vi "slow_control_2_01.vi"() -> ()   [LabVIEW 2018]
uses:
  <vilib>/DAQmx/read.llb/DAQmx Read (Analog 1D DBL NChan 1Samp).vi
  <vilib>/DAQmx/create/channels.llb/DAQmx Create Channel (AI-Voltage-Basic).vi
  <vilib>/DAQmx/miscellaneous.llb/DAQmx Fill In Error Info.vi
  <instrlib>/Lake Shore 335/Lake Shore 335.lvlib
  <instrlib>/CAEN PSM/CAEN PSM.lvlib
panel:
  out "Coldhead":dbl
  out "Heater":dbl
  out "Cycle number":i32
  out "TOBA tester":dbl[][](array[numeric])
  in  "Cycles to execute":dbl=5.0 format="%#_13g"
  out "Moving average Det. P":dbl
  in  "N samples":i32=20
  in  "Allows tabs on \nfront panel":T1(tab)
  in  "Flow meter is AI number:":enum16{"0", "1", "2", "3", "4", "5", "6", "7"}(ring)=enum."3"
  in  "Detector Pressure is AI number:":enum16{"0", "1", "2", "3", "4", "5", "6", "7"}(ring)
  in  "physical channels":tag[](array[tag])=["9207/ai0", "9207/ai1", "9207/ai2", "9207/ai3", "9207/ai4", "9207/ai5", "9207/ai6", "9207/ai7"]
  in  "input terminal configurations":i32[](array[ring]) items=["Default"=-1, "RSE"=10083, "NRSE"=10078, "Differential"=10106, "Pseudodifferential"=12529]
  in  "Heater range":u16(ring) items=["Off", "Low (On)", "Medium", "High"]
  in  "Setpoint (°C)":dbl=-100.0 format="%.1f"
  in  "PID settings":cluster{"P":dbl, "I":dbl, "D":dbl}={"P"=50.0, "I"=20.0, "D"=120.0}
  in  "COM-port LakeShore":refnum<visa-resource-name>
  in  "ID Query":bool=TRUE
  in  "COM-port CAEN 1":refnum<visa-resource-name>
  in  "COM-port CAEN 2":refnum<visa-resource-name>
  out "Heater power (%) 2":cluster{timestamp[], dbl[]}[](graph)
  out "Temp B":dbl
  out "Temp A":dbl
  out "LakeShore readings 2":dbl[](array[numeric])
  out "Raw P (Volt)":dbl[](array[numeric]) format="%0.4f"
  in  "T 20":bool
  in  "T 19":bool
  in  "T 18":bool
  in  "T 17":bool
  in  "T 16":bool
  in  "T 15":bool
  in  "Detector P":bool
  in  "Overpressure threshold":dbl
  in  "Underpressure threshold":dbl
  out "Comm. status":bool
  in  "High Temp threshold":dbl format="%#_13g"
  in  "Low Temp threshold":dbl format="%#_13g"
  in  "Ignore Initialization Errors":bool caption="Ignore init. errors?"
  out "LakeShore status":bool
  out "NI mod1 (P) status":bool
  out "CAEN 1 status":bool
  out "CAEN 2 status":bool
  out "Initialization status":bool
  out "Heater power (%)":cluster{timestamp[], dbl[]}[](graph)
  out "Flow (SLPM)":cluster{timestamp[], dbl[]}[](graph)
  out "Pressure":cluster{timestamp[], dbl[]}[](graph)
  out "Phase Diagram":cluster{"X":dbl, "Y":dbl}[](graph)
  in  "Temp. Channel selector":string(combo)="Average 15 to 20"
  out "Temperature":cluster{timestamp[], dbl[]}[](graph)
  in  "N samples":i32=30
  out "Average Flow (SLPM)":dbl caption="Average Flow (SLPM), of"
  in  "Pause?":bool
  out "Integrated Flow (SL)":dbl
  in  "Reset?":bool
  out "LakeShore readings":dbl[](array[numeric])
  out "Temp. 1":dbl
  out "Temp. 2":dbl
  out "Temp. 3":dbl
  out "Temp. 4":dbl
  out "Temp. 5":dbl
  out "Temp. 6":dbl
  out "Temp. 7":dbl
  out "Temp. 8":dbl
  out "Temp. 9":dbl
  out "Temp. 10":dbl
  out "Temp. 11":dbl
  out "Temp. 12":dbl
  out "Temp. 13":dbl
  out "Temp. 14":dbl
  out "Temp. 15":dbl
  out "Temp. 16":dbl
  out "Temp. 17":dbl
  out "Temp. 18":dbl
  out "Temp. 19":dbl
  out "Temp. 20":dbl
  out "1 to 4":dbl[](array[numeric])
  out "5 to 8":dbl[](array[numeric])
  out "9 to 12":dbl[](array[numeric])
  out "13 to 16":dbl[](array[numeric])
  out "17 to 20":dbl[](array[numeric])
  in  "Temperature Channel selector":string(combo)="Average 15 to 20"
  out "Historical Large Phase Diagram":cluster{dbl[], dbl[]}[](graph)
  out "Large Phase Diagram":cluster{"X":dbl, "Y":dbl}[](graph)
  in  "Temperature Channel selector":string(combo)="Average 15 to 20"
  in  "Set to zero":bool
  out "Bottom gate":dbl(knob) scale=0.0..-3000.0
  out "Top gate":dbl(knob) scale=0.0..3000.0
  in  "Apply Voltage":bool
  in  "VSet (V)":dbl[](array[numeric])
  in  "IMax (uA)":dbl[](array[numeric])
  in  "VMax (V)":dbl[](array[numeric])
  out "Cathode":dbl(knob) scale=0.0..-5000.0
  out "Anode":dbl(knob) scale=0.0..4000.0
  out "PMT 2":dbl(knob) scale=0.0..1000.0
  out "PMT 1":dbl(knob) scale=1.0..1000.0
  out "Vmon (V)":dbl[](array[numeric])
  out "IMon (uA)":dbl[](array[numeric])
  in  "Read V every N cycles":i16=120
  in  "Reset anode":bool
  in  "Kill every Y minutes":i32=10
  in  "Keep off for X seconds":i32=10
  out "?":bool
  out "Killed":bool
  out "Restarted":bool
  out "Anode times":dbl[](array[numeric]) format="%_12f"
  out "Anode times 2":timestamp[](array[timestamp])
  in  "Kill voltage":bool
  in  "stop":bool
  out "Voltages":dbl[](array[numeric])
  out "Started up?":bool
  out "TOBA appended":dbl[][](array[numeric])
  in  "Read T every N cycles":i32=2
  out "Time until next cycle":dbl format="%.3g"
  in  "Time per cycle (s)":i32=2 caption="Time Target (s)"
  # "<- Proof of concept for New/Old T + New P"
  # "PMT 1"
  # "PMT 2"
  # "Anode"
  # "Cathode"
  # "Top gate"
  # "Bottom gate"
  # "Connection settings"
  # "Lakeshore settings"
  # "NI 9207 settings"
  # "Gain (P) (XX.X)"
  # "Reset (I) (XX.X)"
  # "Rate (D) (X.X%)"
  # "Specify inputs:"
  # "Heater tests"
  # "Move to Quick Temp tab ^"
  # "Alarm indicators"
  # "Thresholds"
  # "Alarm conditions"
  # "CAEN 1"
  # "Data"
  # "PMT 1"
  # "PMT 1"
  # "PMT 2"
  # "PMT 2"
  # "Anode"
  # "Anode"
  # "Cathode"
  # "Cathode"
  # "Top gate"
  # "Top gate"
  # "Bottom gate"
  # "Bottom gate"
  # "Settings"
  # "PMT 1"
  # "PMT 1"
  # "PMT 2"
  # "PMT 2"
  # "Anode"
  # "Anode"
  # "Cathode"
  # "Cathode"
  # "Top gate"
  # "Top gate"
  # "Bottom gate"
  # "Bottom gate"
  # "CAEN 2"
  # "PMT 1"
  # "PMT 2"
  # "Anode"
  # "Cathode"
  # "Needle gauges or other displays go here"
  # "Top gate"
  # "Bottom gate"
  # "Time of last reset"
  # "Time of last reactivation"
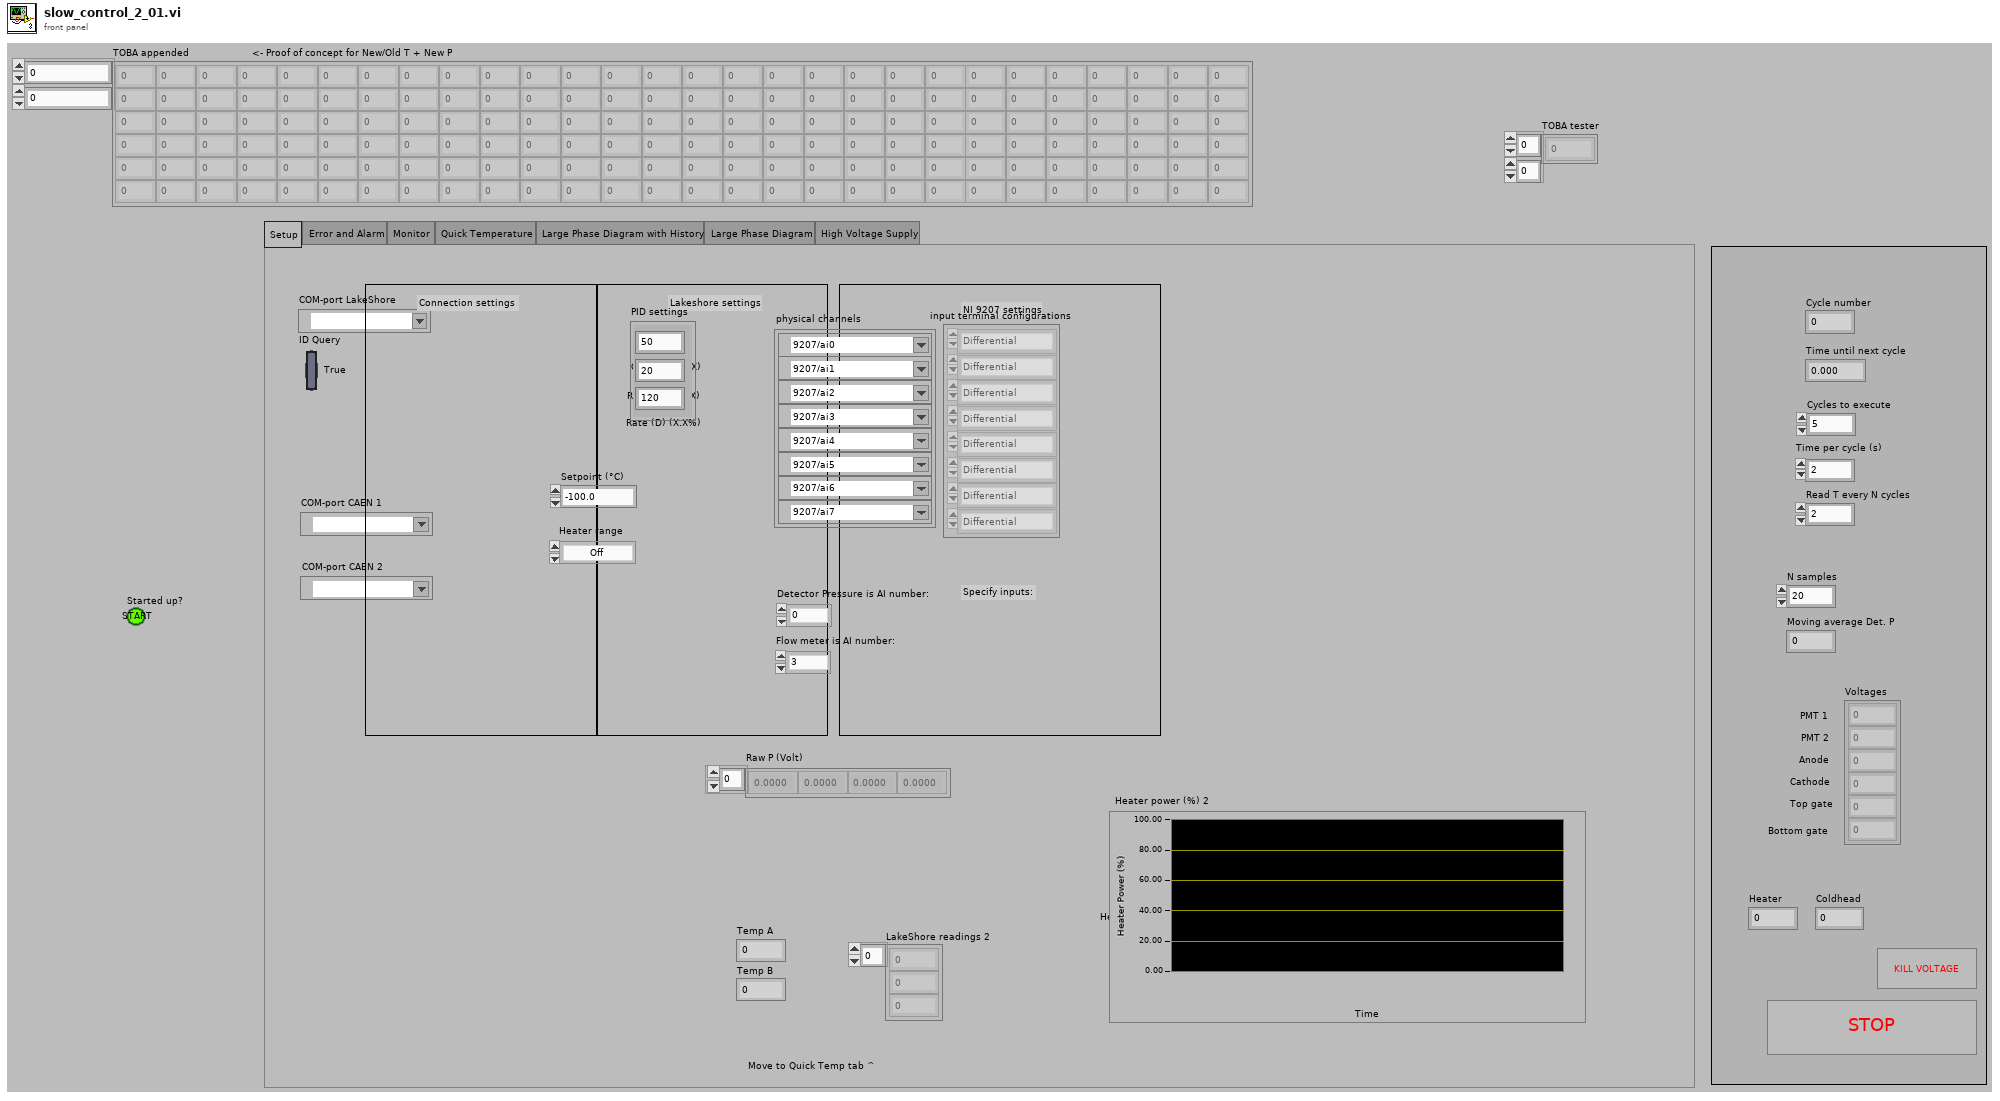
[diagram p1: front panel]
types:
  T1 = enum32{"Setup", "Error and Alarm", "Monitor", "Quick Temperature", "Large Phase Diagram with History", "Large Phase Diagram", "High Voltage Supply"}
  T2 = cluster{"Baud Rate":u32, "Parity":u16, "Data Bits":u16, "Stop Bits":u16, "Flow Control":u16}
  T3 = cluster{"VISA resource name out":refnum<visa-resource-name>, "error out":errorcluster}
  T4 = cluster{"task out":refnum<k21>, "error out":errorcluster}
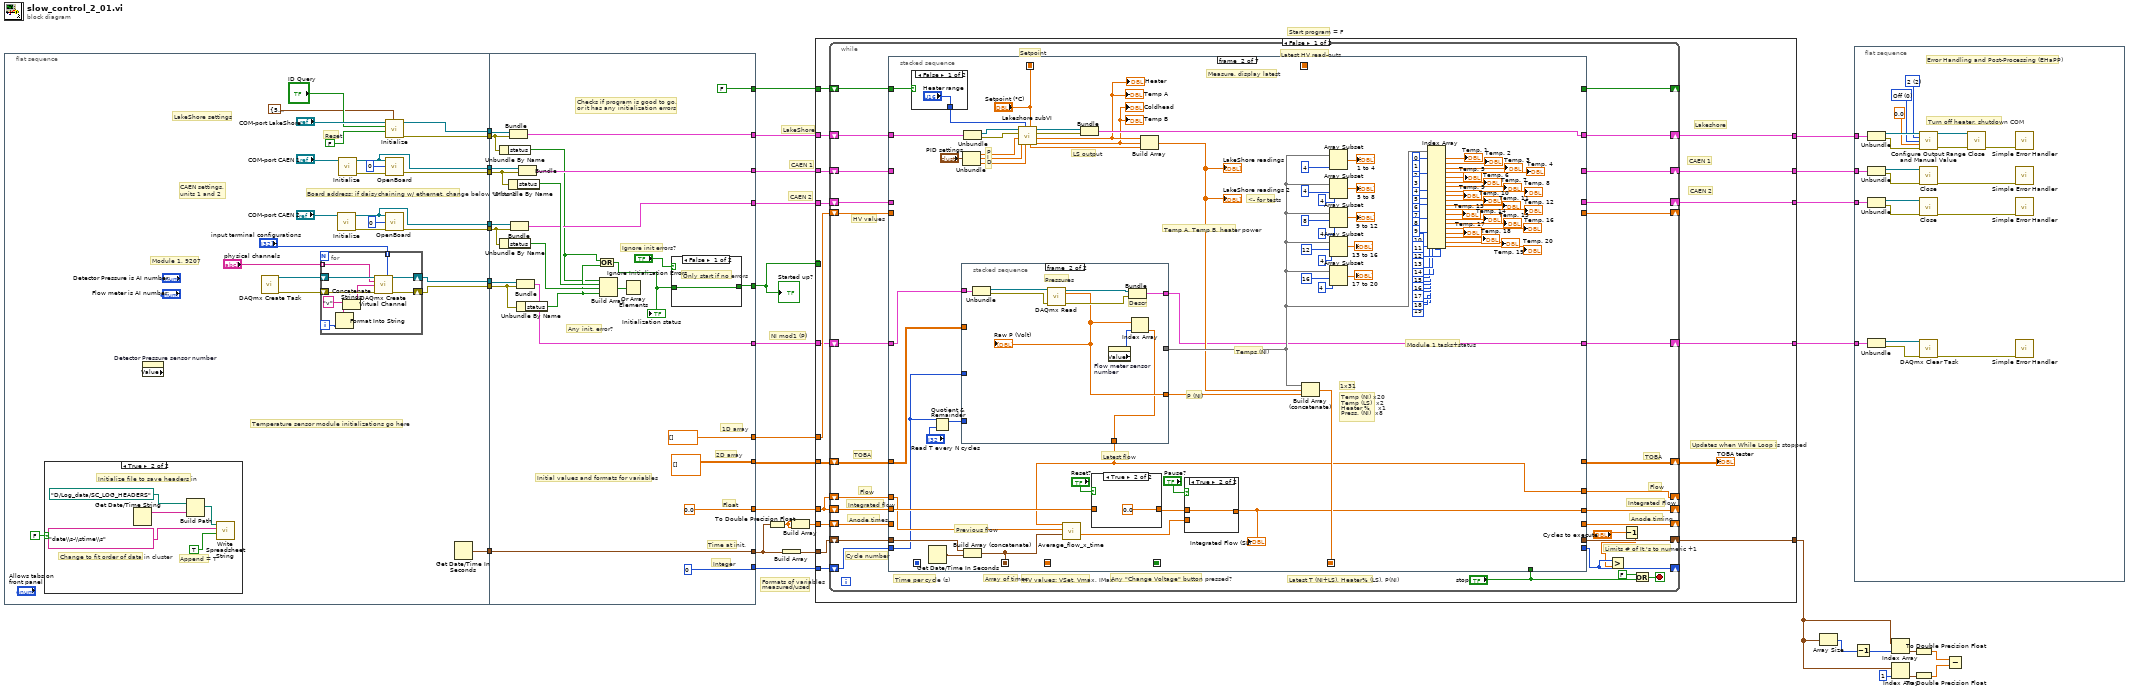
[diagram p0: block diagram]
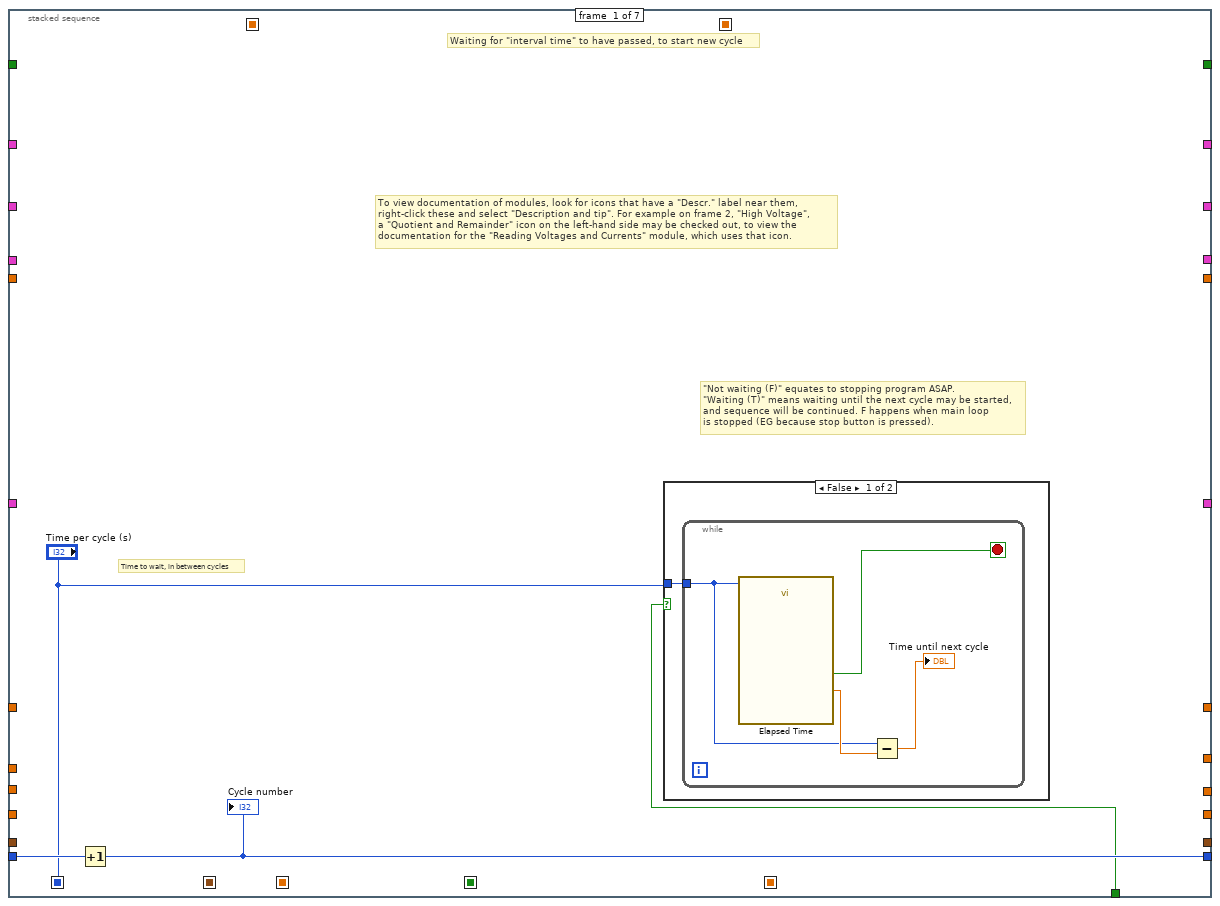
[diagram p2: hidden frame]
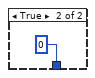
[diagram p4: hidden frame]
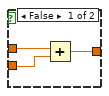
[diagram p6: hidden frame]
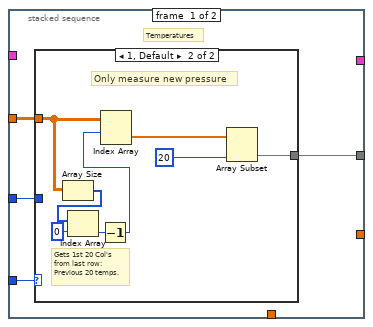
[diagram p7: hidden frame]
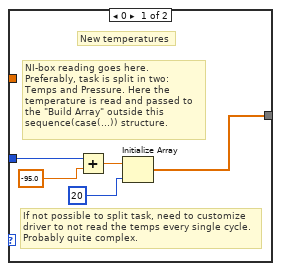
[diagram p8: hidden frame]
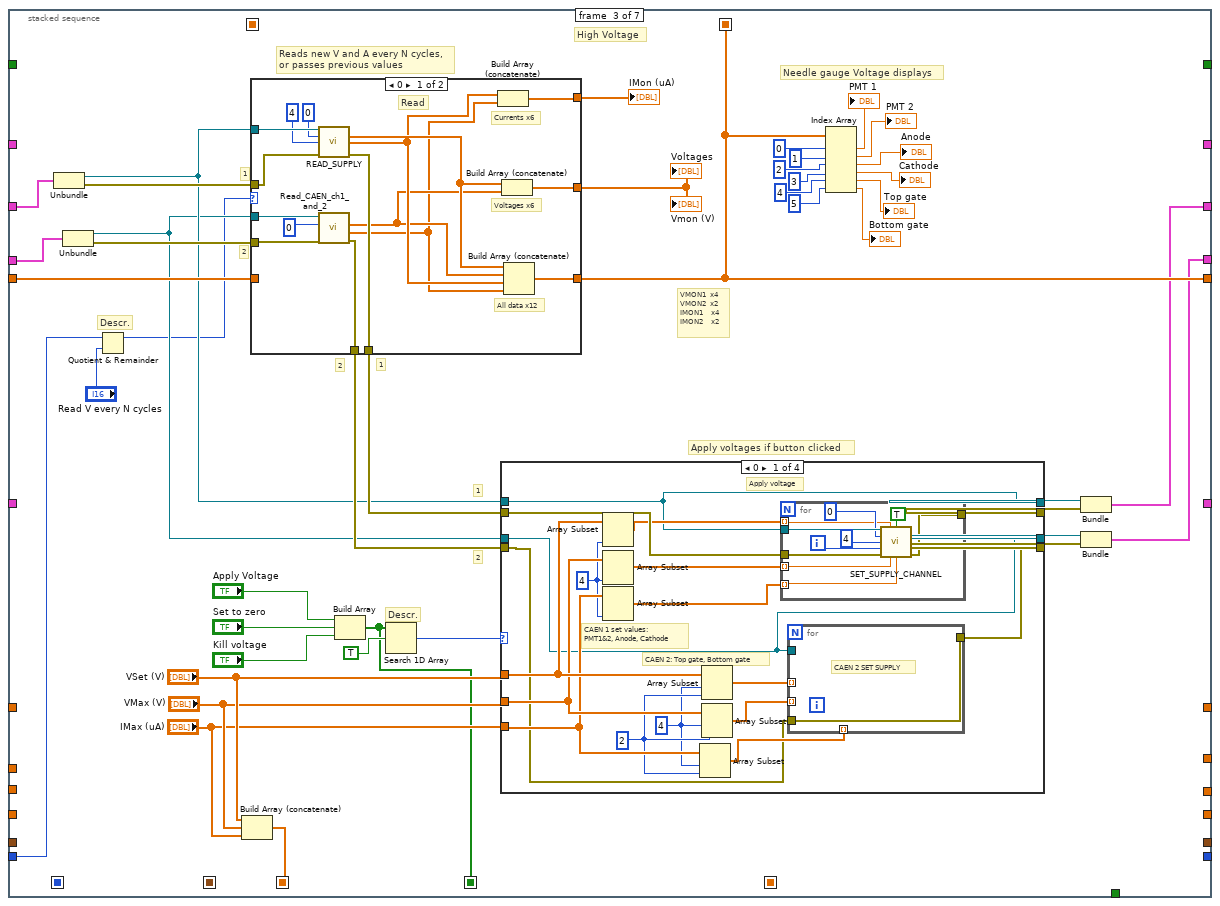
[diagram p9: hidden frame]
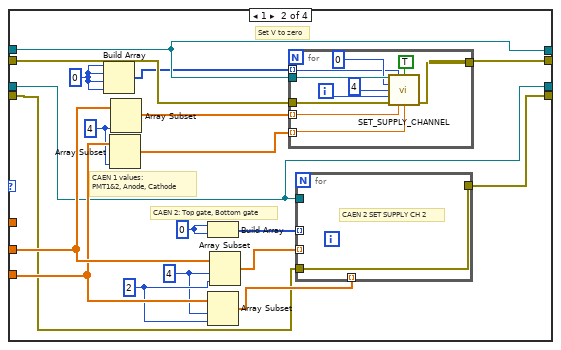
[diagram p10: hidden frame]
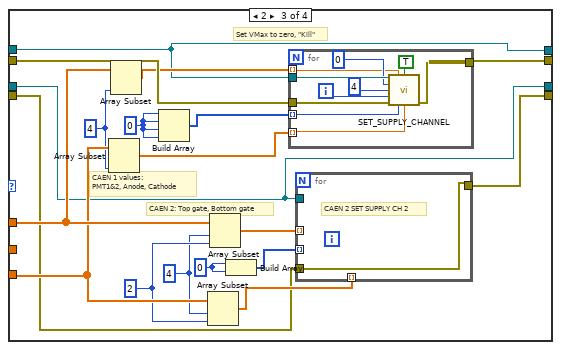
[diagram p11: hidden frame]
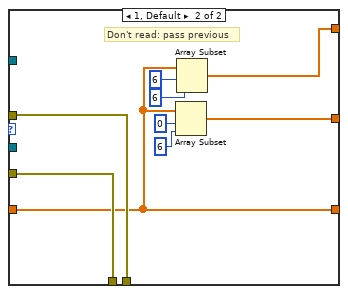
[diagram p13: hidden frame]
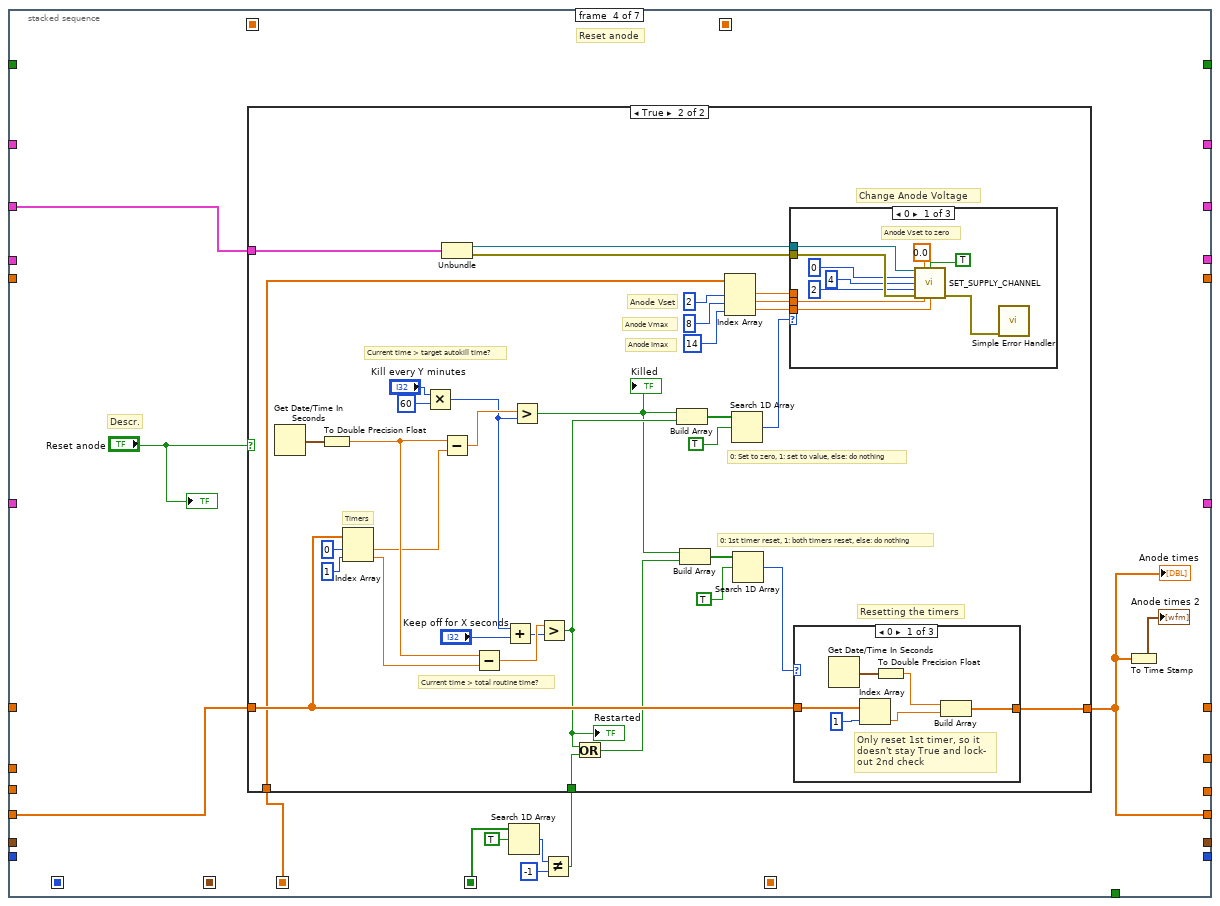
[diagram p14: hidden frame]
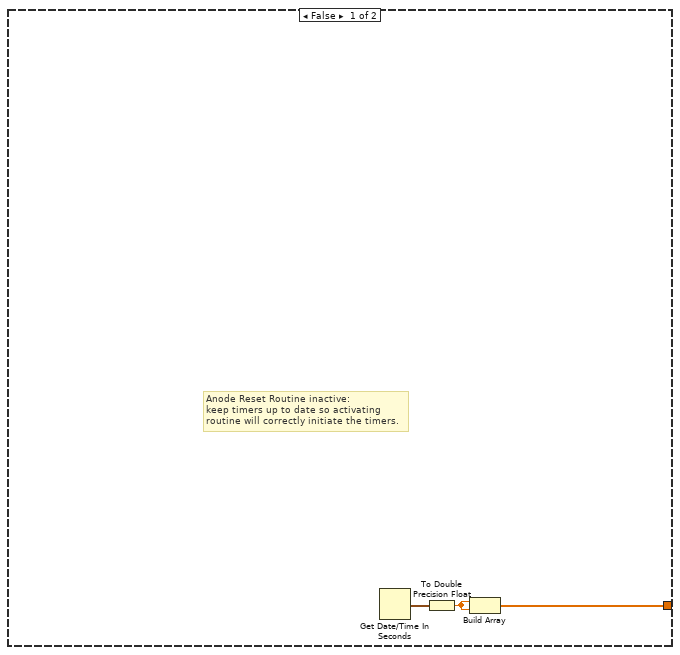
[diagram p15: hidden frame]
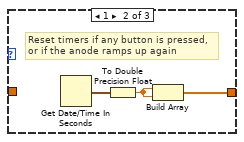
[diagram p16: hidden frame]
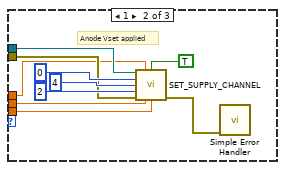
[diagram p18: hidden frame]
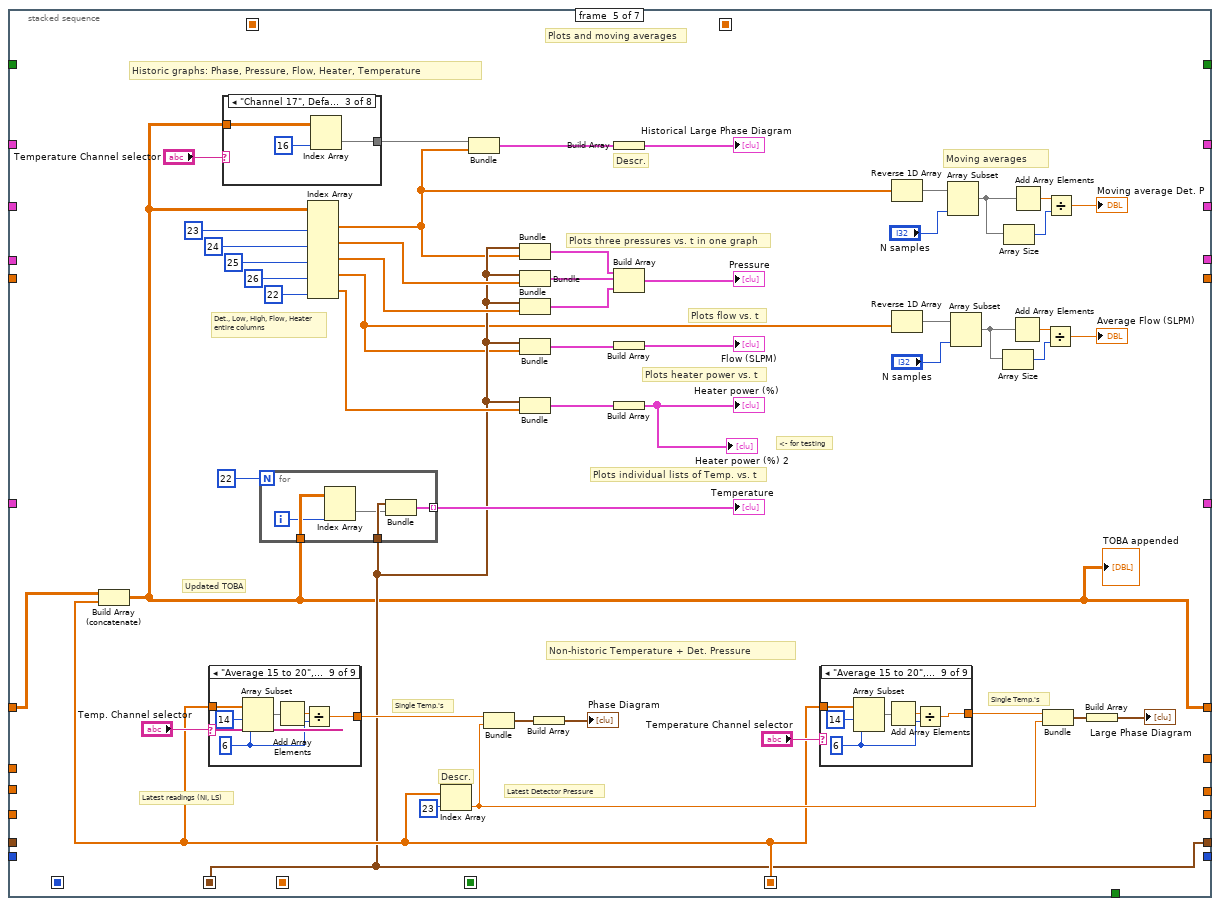
[diagram p20: hidden frame]
diagram:
  # "NI mod1 (P)"
  # "Start program = F"
  # "CAEN 2"
  # "CAEN 1"
  # "LakeShore"
  # "Formats of variables\nmeasured/used"
  n1 = flat-sequence {
    tunnel: [w56] -> w35
    tunnel: [w55] -> w34
    tunnel: [w42] -> w33
    tunnel: [w52] -> w32
    tunnel: [w39] -> w31
    tunnel: [w51] -> w25
    tunnel: [w47] -> w15
    tunnel: [w46] -> w14
    tunnel: [w40] -> w5
    tunnel: w35 -> [w97]
    tunnel: w34 -> [w96]
    tunnel: w33 -> [w94]
    tunnel: w32 -> [w93]
    tunnel: w31 -> [w83]
    tunnel: [w98] -> w12
    tunnel: [0.0] -> w11
    tunnel: [dbl[] []] -> w30
    tunnel: [dbl[][] []] -> w28
    tunnel: [0] -> w29
    tunnel: [w95] -> w27
    tunnel: [w92] -> w26
    tunnel: [w91] -> w10
    tunnel: w25 -> [w91]
    tunnel: w15 -> [w89]
    tunnel: w14 -> [w88]
    tunnel: [w87] -> w13
    tunnel: [FALSE] -> w6
    tunnel: w5 -> [w84]
    tunnel: [w82] -> w4
    frame #0 {
      # "Temperature sensor module initializations go here"
      # "Module 1, 9207"
      # "Board address: if daisychaining w/ ethernet, change below \"0\" to 1"
      # "CAEN settings,\nunits 1 and 2"
      # "Reset"
      # "LakeShore settings"
      n2 = case shown="True" FALSE {
        frame False {
        }
        frame True {
          # "Append = T"
          # "Change to fit order of data in cluster"
          # "Initialize file to save headers in"
          n3 = Get Date/Time String() -> (date string=w74:string)  [unwired: 3 in, 1 out]
          n4 = Build Path(base path=path "D:/Log_data/SC_LOG_HEADERS", name or relative path=w74) -> (appended path=w73:path)
          n5 = call <vilib>:"Write Spreadsheet String.vi"("append to file? (new file:F)"=TRUE, "spreadsheet string"="date\\s-\\stime\\s", "file path (dialog if empty)"=w73) -> ()  [unwired: 7 in, 2 out]
        }
      }
      n6 = property on="Detector Pressure sensor number" class="Enum (strict)" props=["Value"]() -> ()  [unwired: 2 in, 3 out]
      n7 = call <vilib>:"DAQmx Create Task.vi"() -> ("task out"=w38:refnum<k21>, "error out"=w37:errorcluster)  [unwired: 14 in]
      n8 = for {
        shift-right: [w65] -> w40
        shift-left: w38 -> [w64]
        shift-right: [w66] -> w39
        shift-left: w37 -> [w61]
        tunnel: "physical channels" -> [w63] mode=indexing
        tunnel: "input terminal configurations" -> [w62] mode=indexing
        i -> [w68]
        n9 = Format Into String(w68) -> (resulting string=w67:string)  [unwired: 3 in, 1 out]
        n10 = Concatenate Strings("v" ("string"), w67) -> (w60:string)
        n11 = call-poly <vilib>:"DAQmx Create Virtual Channel.vi"("task in"=w64, "input terminal configuration"=w62, "physical channels"=w63, "name to assign"=w60, "error in"=w61) -> ("task out"=w65:refnum<k21>, "error out"=w66:errorcluster)  [unwired: 9 in]
      }
      n12 = call <instrlib>:"Initialize.vi"("VISA resource name"="COM-port CAEN 2") -> ("error out"=w48:errorcluster, "VISA resource name out"=w47:refnum<visa-resource-name>)  [unwired: 9 in]
      n13 = call <instrlib>:"Initialize.vi"("VISA resource name"="COM-port CAEN 1") -> ("error out"=w53:errorcluster, "VISA resource name out"=w42:refnum<visa-resource-name>)  [unwired: 9 in]
      n14 = call <instrlib>:"OpenBoard.vi"("error in (no error)"=w48, "Board Address"=u8 0, "VISA resource name"=w47) -> ("error out"=w46:errorcluster)  [unwired: 7 in, 1 out]
      n15 = call <instrlib>:"Initialize.vi"("Serial Configuration"=T2 {"Baud Rate"=57600, "Parity"=1, "Data Bits"=7, "Stop Bits"=10, "Flow Control"=0}, "Reset (True)"=FALSE ("Reset (LakeShore)"), "ID Query (True)"="ID Query", "VISA resource name"="COM-port LakeShore") -> ("error out"=w55:errorcluster, "VISA resource name out"=w56:refnum<visa-resource-name>)  [unwired: 6 in]
      n16 = call <instrlib>:"OpenBoard.vi"("error in (no error)"=w53, "Board Address"=0, "VISA resource name"=w42) -> ("error out"=w52:errorcluster)  [unwired: 7 in, 1 out]
      n17 = Get Date/Time In Seconds() -> (seconds since 1Jan1904=w51:timestamp)
    }
    frame #1 {
      # "Initial values and formats for variables"
      # "Time at init."
      # "Integer"
      # "2D array"
      # "1D array"
      # "Float"
      # "Checks if program is good to go,\nor it has any initialization errors"
      # "Ignore init errors?"
      # "Any init. error?"
      n18 = Unbundle By Name(w96) -> ("status"=w76:bool)
      n19 = Unbundle By Name(w88) -> ("status"=w90:bool)
      n20 = Unbundle By Name(w93) -> ("status"=w99:bool)
      n21 = Bundle("VISA resource name out"=w97, "error out"=w96) -> (w95:T3)  [unwired: 1 in]
      n22 = Bundle("VISA resource name out"=w89, "error out"=w88) -> (w87:T3)  [unwired: 1 in]
      n23 = Unbundle By Name(w83) -> ("status"=w77:bool)
      n24 = Bundle("task out"=w84, "error out"=w83) -> (w82:T4)  [unwired: 1 in]
      n25 = Bundle("VISA resource name out"=w94, "error out"=w93) -> (w92:T3)  [unwired: 1 in]
      n26 = Or(x=w76, y=w77) -> (x .or. y?=w75:bool)
      "Initialization status" <- w75
      n27 = Build Array(w76, w99, w77, w90) -> (w100:bool[])
      n28 = Or Array Elements(Boolean array=w100) -> ()  [unwired: 1 out]
      n29 = case shown="False" "Ignore Initialization Errors" {
        tunnel: [w101 FALSE] -> w98
        tunnel: w75 -> [w101 _]
        frame False {
          # "Only start if no errors"
        }
        frame True {
          # "Always start program"
        }
      }
    }
  }
  n30 = To Double Precision Float(number=w10) -> (double precision float=w9:dbl)
  n31 = Build Array(w10) -> (w24:timestamp[])
  n32 = Build Array(w9, w9) -> (w8:dbl[])
  n33 = case shown="False" w12 {
    selector: w12 -> [_ w721]
    tunnel: [_ w721] -> _
    tunnel: w30 -> [w112 _]
    tunnel: w29 -> [w119 _]
    tunnel: w28 -> [w118 _]
    tunnel: w27 -> [w113 w719]
    tunnel: w26 -> [w115 w718]
    tunnel: w24 -> [w117 _]
    tunnel: [w116 timestamp[] []] -> w20
    tunnel: w13 -> [w114 w717]
    tunnel: w11 -> [w107 _]
    tunnel: w8 -> [w111 _]
    tunnel: [w109 w719] -> w7
    tunnel: w6 -> [w108 _]
    tunnel: w4 -> [w106 w716]
    tunnel: [w105 w718] -> w3
    tunnel: [w104 w717] -> w2
    tunnel: [w103 w716] -> w1
    frame False {
      # "CAEN 2"
      # "CAEN 1"
      # "Lakeshore"
      # "Updates when While Loop is stopped"
      n34 = while {
        shift-right: [w143] -> _
        shift-left: w119 -> [w148]
        shift-right: [w145] -> w110
        shift-left: w118 -> [w134]
        shift-right: [w135] -> w116
        shift-left: w117 -> [w144]
        shift-right: [w137] -> w105
        shift-left: w115 -> [w126]
        shift-right: [w139] -> _
        shift-left: w112 -> [w142]
        shift-right: [w136] -> w104
        shift-left: w114 -> [w141]
        shift-right: [w138] -> w109
        shift-left: w113 -> [w140]
        shift-right: [w133] -> _
        shift-left: w107 -> [w128]
        shift-right: [w130] -> _
        shift-left: w107 -> [w129]
        shift-right: [w125] -> _
        shift-left: w111 -> [w127]
        shift-right: [w122] -> _
        shift-left: w108 -> [w123]
        shift-right: [w120] -> w103
        shift-left: w106 -> [w121]
        stop <- w146 stop-if-true
        # "Any \"Change Voltage\" button pressed?"
        # "Setpoint"
        # "Anode timing"
        # "Anode times"
        # "Integrated flow"
        # "Flow"
        # "Flow"
        # "Integrated Flow"
        # "TOBA"
        # "Array of times"
        # "Latest HV read-outs"
        # "Time per cycle (s)"
        # "Cycle number"
        # "HV values: VSet, Vmax, IMax"
        # "HV values"
        # "TOBA"
        # "Latest T (NI+LS), Heater% (LS), P(NI)"
        # "Limits # of It.'s to numeric +1"
        n35 = stacked-sequence {
          seq-local: [_ w245 _ _ _ _ _] -> [_ _ _ _ w559 w677 w689]
          seq-local: [_ _ w289 _ _ _ _] -> [_ _ _ w451 _ _ _]
          seq-local: ["Time per cycle (s)" _ _ _ _ _ _] -> [_ _ _ _ _ w673 _]
          seq-local: [_ _ w304 _ _ _ _] -> [_ _ _ _ _ w672 _]
          seq-local: [_ w171 _ _ _ _ _] -> [_ _ _ _ w539 _ _]
          seq-local: [_ _ w283 _ _ _ _] -> [_ _ _ w454 _ _ _]
          seq-local: [_ "Setpoint (°C)" _ _ _ _ _] -> [_ _ _ _ _ w676 _]
          tunnel: [w151 _ _ _ _ _ _] -> w143
          tunnel: "stop" -> [w150 _ _ _ _ _ _]
          tunnel: w148 -> [w152 w159 w318 _ _ _ _]
          tunnel: w134 -> [_ w246 _ _ w566 _ _]
          tunnel: [_ _ _ _ w523 _ _] -> w145
          tunnel: w144 -> [_ w233 _ _ _ _ _]
          tunnel: w126 -> [_ _ w325 w452 _ _ w708]
          tunnel: w142 -> [_ _ w323 _ _ _ _]
          tunnel: w141 -> [_ _ w322 _ _ _ w707]
          tunnel: w140 -> [_ w234 _ _ _ _ w706]
          tunnel: [_ w235 _ _ _ _ _] -> w138
          tunnel: [_ _ w304 _ _ _ _] -> w139
          tunnel: [_ _ w297 _ _ _ _] -> w137
          tunnel: [_ _ w294 _ _ _ _] -> w136
          tunnel: [_ _ _ _ w539 _ _] -> w135
          tunnel: w128 -> [_ w227 _ _ _ _ _]
          tunnel: [_ w228 _ _ _ _ _] -> w133
          tunnel: [_ w169 _ _ _ _ _] -> w130
          tunnel: w129 -> [_ w168 _ _ _ _ _]
          tunnel: w127 -> [_ _ _ w453 _ _ _]
          tunnel: [_ _ _ w447 _ _ _] -> w125
          tunnel: w123 -> [_ w163 _ _ _ _ _]
          tunnel: [_ _ _ _ _ _ FALSE] -> w122
          tunnel: w121 -> [_ w161 _ _ _ _ w704]
          tunnel: [_ w160 _ _ _ _ _] -> w120
          frame #0 {
            # "To view documentation of modules, look for icons that have a \"Descr.\" label near them,\nright-click these and select \"Description and tip\". For example on frame 2, \"High Voltage\",\na \"Quotient and Remainder\" icon on the left-hand side may be checked out, to view the\ndocumentation for the \"Reading Voltages and Currents\" module, which uses that icon."
            # "Time to wait, in between cycles"
            # "\"Not waiting (F)\" equates to stopping program ASAP.\n\"Waiting (T)\" means waiting until the next cycle may be started,\nand sequence will be continued. F happens when main loop \nis stopped (EG because stop button is pressed)."
            # "Waiting for \"interval time\" to have passed, to start new cycle"
            n36 = Increment(x=w152) -> (x+1=w151:i32)
            "Cycle number" <- w151
            n37 = case shown="False" w150 {
              tunnel: "Time per cycle (s)" -> [w153 _]
              frame False {
                n38 = while {
                  tunnel: w153 -> [w155]
                  stop <- w157 stop-if-true
                  n39 = call "Elapsed Time"("Time Target (s)"=w155) -> ("Elapsed Time (s)"=w156:dbl, "Time has Elapsed"=w157:bool)  [unwired: 11 in, 6 out]
                  n40 = Subtract(x=w155, y=w156) -> (x-y=→"Time until next cycle":dbl)
                }
              }
              frame True {
              }
            }
          }
          frame #1 {
            # "Previous flow"
            # "Latest flow"
            # "Module 1 tasks+status"
            # "<- for tests"
            # "P (NI)"
            # "Temps (NI)"
            # "1x31"
            # "LS output"
            # "Temp (NI) x20\nTemp (LS)  x2\nHeater %    x1\nPress. (NI)  x8"
            # "Temp A, Temp B, heater power"
            # "P\nI\nD"
            # "Measure, display latest"
            n41 = case shown="False" w163 {
              tunnel: ["Heater range" 0] -> w238
              frame False {
              }
              frame True {
              }
            }
            n42 = Get Date/Time In Seconds() -> (seconds since 1Jan1904=w232:timestamp)
            n43 = Quotient & Remainder(x=w159, y="Read T every N cycles") -> (x-y*floor(x/y)=w247:i32)  [unwired: 1 out]
            n44 = stacked-sequence {
              tunnel: w247 -> [w260 _]
              tunnel: [w259 _] -> w170
              tunnel: [_ w275] -> w231
              tunnel: w246 -> [w258 _]
              tunnel: w159 -> [w257 _]
              tunnel: [_ w274] -> w169
              tunnel: w161 -> [_ w282]
              tunnel: [_ w277] -> w160
              frame #0 {
                # "Temperatures"
                n45 = case shown="1, Default" w260 {
                  tunnel: w258 -> [_ w270]
                  tunnel: [w263 w266] -> w259
                  tunnel: w257 -> [w262 _]
                  frame 0 {
                    # "If not possible to split task, need to customize\ndriver to not read the temps every single cycle.\nProbably quite complex."
                    # "NI-box reading goes here.\nPreferably, task is split in two: \nTemps and Pressure. Here the \ntemperature is read and passed to \nthe \"Build Array\" outside this \nsequence(case(...)) structure."
                    # "New temperatures"
                    n46 = Add(x=w262, y=-95.0 ("element")) -> (x+y=w265:dbl)
                    n47 = Initialize Array(w265, 20) -> (w263:dbl[])
                  }
                  frame 1, Default {
                    # "Gets 1st 20 Col's\nfrom last row:\nPrevious 20 temps."
                    # "Only measure new pressure"
                    n48 = Array Size(array=w270) -> (size(s)=w272:i32[])
                    n49 = Index Array(array=w272, index=0) -> (element=w273:i32)
                    n50 = Decrement(x=w273) -> (x-1=w269:i32)
                    n51 = Index Array(array=w270, index (row)=w269) -> (element=w268:dbl[])  [unwired: 1 in]
                    n52 = Array Subset(array=w268, length=20) -> (w266:dbl[])  [unwired: 1 in]
                  }
                }
              }
              frame #1 {
                # "Descr"
                # "Pressures"
                n53 = Unbundle(w282) -> ("task out"=w281:refnum<k21>, "error out"=w280:errorcluster)
                n54 = call-poly <vilib>:"DAQmx Read.vi"("task/channels in"=w281, "error in"=w280) -> ("task out"=w279:refnum<k21>, "data"=w275:dbl[], "error out"=w278:errorcluster)  [unwired: 11 in]
                "Raw P (Volt)" <- w275
                n55 = property on="Flow meter sensor number" class="Enum (strict)"() -> ("Value"=w276:enum16{"0", "1", "2", "3", "4", "5", "6", "7"})  [unwired: 2 in, 2 out]
                n56 = Bundle("task out"=w279, "error out"=w278) -> (w277:T4)  [unwired: 1 in]
                n57 = Index Array(array=w275, index=w276) -> (element=w274:dbl)
              }
            }
            n58 = Unbundle("PID settings") -> ("P"=w241:dbl, "I"=w240:dbl, "D"=w239:dbl)
            n59 = Build Array (concatenate)(w233, w232) -> (w171:timestamp[])
            n60 = Unbundle(w234) -> ("VISA resource name out"=w243:refnum<visa-resource-name>, "error out"=w242:errorcluster)
            n61 = call "Lakeshore subVI.vi"("Setpoint"="Setpoint (°C)", "Rate (D) (X.X %)"=w239, "Range"=w238, "Reset (I) (XX.X)"=w240, "Gain (P) (XX.X)"=w241, "error in (no error)"=w242, "VISA resource name"=w243) -> ("Input B"=w166:dbl, "Input A"=w167:dbl, "error out"=w236:errorcluster, "VISA resource name out"=w237:refnum<visa-resource-name>, "Heater 1 (%)"=w165:dbl)
            "Temp A" <- w167
            "Temp B" <- w166
            "Coldhead" <- w166
            "Heater" <- w167
            n62 = call "Average_flow_x_time.vi"("Array of timestamps"=w171, "Previous Flow"=w168, "Latest Flow"=w169) -> ("Volume (SL)"=w158:dbl)  [unwired: 8 in]
            n63 = Bundle("VISA resource name out"=w237, "error out"=w236) -> (w235:T3)  [unwired: 1 in]
            n64 = case shown="True" "Reset?" {
              tunnel: w227 -> [w251 _]
              tunnel: [w251 0.0] -> w226
              frame False {
              }
              frame True {
              }
            }
            n65 = Build Array(w167, w166, w165) -> (w164:dbl[])
            "LakeShore readings" <- w164
            "LakeShore readings 2" <- w164
            n66 = case shown="True" "Pause?" {
              tunnel: w158 -> [w255 _]
              tunnel: w226 -> [w254 w256]
              tunnel: [w253 w256] -> w228
              frame False {
                n67 = Add(x=w254, y=w255) -> (x+y=w253:dbl)
              }
              frame True {
              }
            }
            "Integrated Flow (SL)" <- w228
            n68 = Build Array (concatenate)(w170, w164, w231) -> (w245:dbl[])
            n69 = Array Subset(array=w170, length=4) -> (→"1 to 4":dbl[])  [unwired: 1 in]
            n70 = Array Subset(array=w170, index=4, length=4 ("index")) -> (→"5 to 8":dbl[])
            n71 = Array Subset(array=w170, index=8, length=4 ("index")) -> (→"9 to 12":dbl[])
            n72 = Array Subset(array=w170, index=12, length=4 ("index")) -> (→"13 to 16":dbl[])
            n73 = Array Subset(array=w170, index=16, length=4 ("index")) -> (→"17 to 20":dbl[])
            n74 = Index Array(array=w170, index #1=0, index #2=1, index #3=2, index #4=3, index #5=4, index #6=5, index #7=6, index #8=7, index #9=8, index #10=9, index #11=10, index #12=11, index #13=12, index #14=13, index #15=14, index #16=15, index #17=16, index #18=17, index #19=18, index #20=19) -> (element #1=→"Temp. 1":dbl, element #2=→"Temp. 2":dbl, element #3=→"Temp. 3":dbl, element #4=→"Temp. 4":dbl, element #5=→"Temp. 5":dbl, element #6=→"Temp. 6":dbl, element #7=→"Temp. 7":dbl, element #8=→"Temp. 8":dbl, element #9=→"Temp. 9":dbl, element #10=→"Temp. 10":dbl, element #11=→"Temp. 11":dbl, element #12=→"Temp. 12":dbl, element #13=→"Temp. 13":dbl, element #14=→"Temp. 14":dbl, element #15=→"Temp. 15":dbl, element #16=→"Temp. 16":dbl, element #17=→"Temp. 17":dbl, element #18=→"Temp. 18":dbl, element #19=→"Temp. 19":dbl, element #20=→"Temp. 20":dbl)
          }
          frame #2 {
            # "Apply voltages if button clicked"
            # "2"
            # "1"
            # "Descr."
            # "Descr."
            # "VMON1  x4 \nVMON2  x2\nIMON1    x4\nIMON2    x2"
            # "Needle gauge Voltage displays"
            # "1"
            # "2"
            # "1"
            # "2"
            # "Reads new V and A every N cycles,\nor passes previous values"
            # "High Voltage"
            n75 = Unbundle(w325) -> ("VISA resource name out"=w300:refnum<visa-resource-name>, "error out"=w324:errorcluster)
            n76 = Unbundle(w322) -> ("VISA resource name out"=w299:refnum<visa-resource-name>, "error out"=w321:errorcluster)
            n77 = Quotient & Remainder(x=w318, y="Read V every N cycles") -> (x-y*floor(x/y)=w284:i32)  [unwired: 1 out]
            n78 = Build Array (concatenate)("VSet (V)", "VMax (V)", "IMax (uA)") -> (w289:dbl[])
            n79 = case shown="0" w284 {
              tunnel: w300 -> [w434 _]
              tunnel: w324 -> [w433 w442]
              tunnel: w323 -> [_ w438]
              tunnel: w299 -> [w424 _]
              tunnel: w321 -> [w422 w443]
              tunnel: [w421 w443] -> w301
              tunnel: [w430 w442] -> w302
              tunnel: [w429 w438] -> w304
              tunnel: [w427 w439] -> w320
              tunnel: [w425 w435] -> w319
              frame 0 {
                # "All data x12"
                # "Voltages x6"
                # "Currents x6"
                # "Read"
                n80 = call "READ_SUPPLY.vi"("VISA resource name"=w434, "Board address"=u8 0, "NChannels"=u8 4, "error in (no error)"=w433) -> ("VMon values (V)"=w428:dbl[], "IMon values (uA)"=w426:dbl[], "error out"=w430:errorcluster)  [unwired: 9 in]
                n81 = call "Read_CAEN_ch1_and_2.vi"("VISA resource name in"=w424, "Board address"=u8 0, "error in"=w422) -> ("VMon values (V)"=w420:dbl[], "IMon values (uA)"=w419:dbl[], "error out"=w421:errorcluster)  [unwired: 4 in, 1 out]
                n82 = Build Array (concatenate)(w426, w419) -> (w425:dbl[])
                n83 = Build Array (concatenate)(w428, w420) -> (w427:dbl[])
                n84 = Build Array (concatenate)(w428, w420, w426, w419) -> (w429:dbl[])
              }
              frame 1, Default {
                # "Don't read: pass previous"
                n85 = Array Subset(array=w438, index=0, length=6) -> (w439:dbl[])
                n86 = Array Subset(array=w438, index=6, length=6) -> (w435:dbl[])
              }
            }
            "Voltages" <- w320
            "Vmon (V)" <- w320
            "IMon (uA)" <- w319
            n87 = Build Array("Apply Voltage", "Set to zero", "Kill voltage") -> (w283:bool[])
            n88 = Search 1D Array(1D array=w283, element=TRUE) -> (index of element=w303:i32)  [unwired: 1 in]
            n89 = case shown="0" w303 {
              tunnel: w302 -> [w343 w373 w403 w415]
              tunnel: w301 -> [w329 w362 w392 w417]
              tunnel: w300 -> [w339 w370 w400 w418]
              tunnel: w299 -> [w327 w360 w390 w416]
              tunnel: [w340 w371 w401 w415] -> w293
              tunnel: [w339 w370 w400 w418] -> w298
              tunnel: [w326 w359 w389 w417] -> w295
              tunnel: [w327 w360 w390 w416] -> w296
              tunnel: "VSet (V)" -> [w337 _ w398 _]
              tunnel: "VMax (V)" -> [w336 w368 _ _]
              tunnel: "IMax (uA)" -> [w335 w367 w397 _]
              frame 0 {
                w328 = 4 ("length")
                w333 = 2 ("length")
                w334 = 4 ("length")
                # "CAEN 2: Top gate, Bottom gate"
                # "CAEN 1 set values:\nPMT1&2, Anode, Cathode"
                # "Apply voltage"
                n90 = Array Subset(array=w337, length=w334) -> (w342:dbl[])  [unwired: 1 in]
                n91 = Array Subset(array=w336, length=w334) -> (w341:dbl[])  [unwired: 1 in]
                n92 = Array Subset(array=w335, length=w334) -> (w338:dbl[])  [unwired: 1 in]
                n93 = Array Subset(array=w335, index=w328, length=w333) -> (w330:dbl[])
                n94 = Array Subset(array=w337, index=w328, length=w333) -> (w332:dbl[])
                n95 = Array Subset(array=w336, index=w328, length=w333) -> (w331:dbl[])
                n96 = for {
                  tunnel: w339 -> [w353]
                  tunnel: w343 -> [w352]
                  tunnel: w342 -> [w349] mode=indexing
                  tunnel: w341 -> [w347] mode=indexing
                  tunnel: w338 -> [w346] mode=indexing
                  tunnel: [w345] -> w340
                  i -> [w354]
                  n97 = call "SET_SUPPLY_CHANNEL.vi"("VISA resource name"=w353, "Voltage Level (0.0 V)"=w349, "Enable (OFF)"=TRUE, "Board address"=u8 0, "NChannels"=u8 4, "Channel (0)"=w354, "error in (no error)"=w352, "Voltage Max (0.0 V)"=w347, "Current Limit (0.00 uA)"=w346) -> ("error out"=w345:errorcluster)  [unwired: 6 in]
                }
                n98 = for {
                  tunnel: w327 -> [_]
                  tunnel: w329 -> [w344]
                  tunnel: w332 -> [_] mode=indexing
                  tunnel: w331 -> [_] mode=indexing
                  tunnel: w330 -> [_] mode=indexing
                  tunnel: [w344] -> w326
                  # "CAEN 2 SET SUPPLY"
                }
              }
              frame 1 {
                w355 = 0 ("length")
                w357 = 0 ("length")
                w361 = 4 ("length")
                w365 = 2 ("length")
                w366 = 4 ("length")
                # "CAEN 2: Top gate, Bottom gate"
                # "CAEN 1 values:\nPMT1&2, Anode, Cathode"
                # "Set V to zero"
                n99 = Build Array(w357, w357, w357, w357) -> (w358:i32[])
                n100 = Array Subset(array=w367, length=w366) -> (w369:dbl[])  [unwired: 1 in]
                n101 = Array Subset(array=w368, length=w366) -> (w372:dbl[])  [unwired: 1 in]
                n102 = Build Array(w355, w355) -> (w356:i32[])
                n103 = Array Subset(array=w367, index=w361, length=w365) -> (w363:dbl[])
                n104 = Array Subset(array=w368, index=w361, length=w365) -> (w364:dbl[])
                n105 = for {
                  tunnel: w370 -> [w383]
                  tunnel: w373 -> [w382]
                  tunnel: w358 -> [w379] mode=indexing
                  tunnel: w372 -> [w377] mode=indexing
                  tunnel: w369 -> [w376] mode=indexing
                  tunnel: [w375] -> w371
                  i -> [w384]
                  n106 = call "SET_SUPPLY_CHANNEL.vi"("VISA resource name"=w383, "Voltage Level (0.0 V)"=w379, "Enable (OFF)"=TRUE, "Board address"=u8 0, "NChannels"=u8 4, "Channel (0)"=w384, "error in (no error)"=w382, "Voltage Max (0.0 V)"=w377, "Current Limit (0.00 uA)"=w376) -> ("error out"=w375:errorcluster)  [unwired: 6 in]
                }
                n107 = for {
                  tunnel: w360 -> [_]
                  tunnel: w362 -> [w374]
                  tunnel: w356 -> [_] mode=indexing
                  tunnel: w364 -> [_] mode=indexing
                  tunnel: w363 -> [_] mode=indexing
                  tunnel: [w374] -> w359
                  # "CAEN 2 SET SUPPLY CH 2"
                }
              }
              frame 2 {
                w386 = 0 ("length")
                w388 = 0 ("length")
                w391 = 4 ("length")
                w395 = 2 ("length")
                w396 = 4 ("length")
                # "CAEN 2: Top gate, Bottom gate"
                # "CAEN 1 values:\nPMT1&2, Anode, Cathode"
                # "Set VMax to zero, \"Kill\""
                n108 = Array Subset(array=w397, length=w396) -> (w399:dbl[])  [unwired: 1 in]
                n109 = Array Subset(array=w398, length=w396) -> (w402:dbl[])  [unwired: 1 in]
                n110 = Build Array(w388, w388, w388, w388) -> (w387:i32[])
                n111 = Array Subset(array=w397, index=w391, length=w395) -> (w393:dbl[])
                n112 = Array Subset(array=w398, index=w391, length=w395) -> (w394:dbl[])
                n113 = Build Array(w386, w386) -> (w385:i32[])
                n114 = for {
                  tunnel: w400 -> [w413]
                  tunnel: w403 -> [w412]
                  tunnel: w402 -> [w409] mode=indexing
                  tunnel: w387 -> [w407] mode=indexing
                  tunnel: w399 -> [w406] mode=indexing
                  tunnel: [w405] -> w401
                  i -> [w414]
                  n115 = call "SET_SUPPLY_CHANNEL.vi"("VISA resource name"=w413, "Voltage Level (0.0 V)"=w409, "Enable (OFF)"=TRUE, "Board address"=u8 0, "NChannels"=u8 4, "Channel (0)"=w414, "error in (no error)"=w412, "Voltage Max (0.0 V)"=w407, "Current Limit (0.00 uA)"=w406) -> ("error out"=w405:errorcluster)  [unwired: 6 in]
                }
                n116 = for {
                  tunnel: w390 -> [_]
                  tunnel: w392 -> [w404]
                  tunnel: w394 -> [_] mode=indexing
                  tunnel: w385 -> [_] mode=indexing
                  tunnel: w393 -> [_] mode=indexing
                  tunnel: [w404] -> w389
                  # "CAEN 2 SET SUPPLY CH 2"
                }
              }
              frame 3, Default {
                # "\"Executes\" if none of the three buttons have been clicked"
                # "Do nothing"
              }
            }
            n117 = Index Array(array=w304, index #1=0 ("index"), index #2=1 ("index"), index #3=2 ("index"), index #4=3 ("index"), index #5=4 ("index"), index #6=5 ("index")) -> (element #1=→"PMT 1":dbl, element #2=→"PMT 2":dbl, element #3=→"Anode":dbl, element #4=→"Cathode":dbl, element #5=→"Top gate":dbl, element #6=→"Bottom gate":dbl)
            n118 = Bundle("VISA resource name out"=w298, "error out"=w293) -> (w297:T3)  [unwired: 1 in]
            n119 = Bundle("VISA resource name out"=w296, "error out"=w295) -> (w294:T3)  [unwired: 1 in]
          }
          frame #3 {
            # "Descr."
            # "Reset anode"
            n120 = Search 1D Array(1D array=w454, element=TRUE) -> (index of element=w445:i32)  [unwired: 1 in]
            n121 = Not Equal?(x=w445, y=-1) -> (x != y?=w450:bool)
            n122 = case shown="True" "Reset anode" {
              tunnel: w453 -> [_ w477]
              tunnel: w452 -> [_ w489]
              tunnel: w451 -> [_ w458]
              tunnel: w450 -> [_ w479]
              tunnel: [w455 w459] -> w447
              frame False {
                # "Anode Reset Routine inactive:\nkeep timers up to date so activating\nroutine will correctly initiate the timers."
                n123 = Get Date/Time In Seconds() -> (seconds since 1Jan1904=w457:timestamp)
                n124 = To Double Precision Float(number=w457) -> (double precision float=w456:dbl)
                n125 = Build Array(w456, w456) -> (w455:dbl[])
              }
              frame True {
                # "0: 1st timer reset, 1: both timers reset, else: do nothing"
                # "Timers"
                # "0: Set to zero, 1: set to value, else: do nothing"
                # "Resetting the timers"
                # "Change Anode Voltage"
                # "Anode Imax"
                # "Anode Vmax"
                # "Anode Vset"
                # "Current time > total routine time?"
                # "Current time > target autokill time?"
                n126 = Get Date/Time In Seconds() -> (seconds since 1Jan1904=w491:timestamp)
                n127 = To Double Precision Float(number=w491) -> (double precision float=w472:dbl)
                n128 = Index Array(array=w477, index #1=0 ("index"), index #2=1 ("index")) -> (element #1=w471:dbl, element #2=w473:dbl)
                n129 = Multiply(x="Kill every Y minutes", y=60) -> (x*y=w469:i32)
                n130 = Unbundle(w489) -> ("VISA resource name out"=w488:refnum<visa-resource-name>, "error out"=w487:errorcluster)
                n131 = Subtract(x=w472, y=w471) -> (x-y=w470:dbl)
                n132 = Subtract(x=w472, y=w473) -> (x-y=w461:dbl)
                n133 = Add(x=w469, y="Keep off for X seconds") -> (x+y=w460:i32)
                n134 = Greater?(x=w470, y=w469) -> (0:w463:bool)
                "Killed" <- w463
                n135 = Greater?(x=w461, y=w460) -> (0:w464:bool)
                "Restarted" <- w464
                n136 = Or(x=w464, y=w479) -> (x .or. y?=w467:bool)
                n137 = Build Array(w463, w464) -> (w481:bool[])
                n138 = Build Array(w463, w467) -> (w468:bool[])
                n139 = Index Array(array=w458, index #1=2 ("index"), index #2=8 ("index"), index #3=14 ("index")) -> (element #1=w484:dbl, element #2=w482:dbl, element #3=w483:dbl)
                n140 = Search 1D Array(1D array=w481, element=TRUE) -> (index of element=w480:i32)  [unwired: 1 in]
                n141 = Search 1D Array(1D array=w468, element=TRUE) -> (index of element=w465:i32)  [unwired: 1 in]
                n142 = case shown="0" w480 {
                  tunnel: w484 -> [_ w516 _]
                  tunnel: w482 -> [w504 w515 _]
                  tunnel: w483 -> [w506 w514 _]
                  tunnel: w488 -> [w512 w519 _]
                  tunnel: w487 -> [w511 w518 _]
                  frame 0 {
                    # "Anode Vset to zero"
                    n143 = call "SET_SUPPLY_CHANNEL.vi"("VISA resource name"=w512, "Voltage Level (0.0 V)"=0.0, "Enable (OFF)"=TRUE, "Board address"=u8 0, "NChannels"=u8 4, "Channel (0)"=u8 2, "error in (no error)"=w511, "Voltage Max (0.0 V)"=w504, "Current Limit (0.00 uA)"=w506) -> ("error out"=w505:errorcluster)  [unwired: 6 in]
                    n144 = call <vilib>:"Simple Error Handler.vi"("error in (no error)"=w505) -> ()  [unwired: 4 in, 5 out]
                  }
                  frame 1 {
                    # "Anode Vset applied"
                    n145 = call "SET_SUPPLY_CHANNEL.vi"("VISA resource name"=w519, "Voltage Level (0.0 V)"=w516, "Enable (OFF)"=TRUE, "Board address"=u8 0, "NChannels"=u8 4, "Channel (0)"=u8 2, "error in (no error)"=w518, "Voltage Max (0.0 V)"=w515, "Current Limit (0.00 uA)"=w514) -> ("error out"=w513:errorcluster)  [unwired: 6 in]
                    n146 = call <vilib>:"Simple Error Handler.vi"("error in (no error)"=w513) -> ()  [unwired: 4 in, 5 out]
                  }
                  frame 2, Default {
                    # "Do nothing"
                  }
                }
                n147 = case shown="0" w465 {
                  tunnel: [w493 w499 w502] -> w459
                  tunnel: w477 -> [w497 _ w502]
                  frame 0 {
                    # "Only reset 1st timer, so it\ndoesn't stay True and lock-\nout 2nd check"
                    n148 = Get Date/Time In Seconds() -> (seconds since 1Jan1904=w496:timestamp)
                    n149 = Index Array(array=w497, index=1) -> (element=w494:dbl)
                    n150 = To Double Precision Float(number=w496) -> (double precision float=w495:dbl)
                    n151 = Build Array(w495, w494) -> (w493:dbl[])
                  }
                  frame 1 {
                    # "Reset timers if any button is pressed,\nor if the anode ramps up again"
                    n152 = Get Date/Time In Seconds() -> (seconds since 1Jan1904=w501:timestamp)
                    n153 = To Double Precision Float(number=w501) -> (double precision float=w500:dbl)
                    n154 = Build Array(w500, w500) -> (w499:dbl[])
                  }
                  frame 2, Default {
                    # "Time difference grows \nlarger for now"
                  }
                }
              }
            }
            "Anode times" <- w447
            n155 = To Time Stamp(1:w447) -> (0:→"Anode times 2":timestamp[])
            "?" <- "Reset anode"
          }
          frame #4 {
            # "<- for testing"
            # "Descr."
            # "Moving averages"
            # "Plots heater power vs. t"
            # "Historic graphs: Phase, Pressure, Flow, Heater, Temperature"
            # "Plots flow vs. t"
            # "Plots three pressures vs. t in one graph"
            # "Non-historic Temperature + Det. Pressure"
            # "Det., Low, High, Flow, Heater\nentire columns"
            # "Latest readings (NI, LS)"
            # "Single Temp.'s"
            # "Single Temp.'s"
            # "Updated TOBA"
            # "Descr."
            # "Latest Detector Pressure"
            # "Plots individual lists of Temp. vs. t"
            # "Plots and moving averages"
            n156 = Build Array (concatenate)(w566, w559) -> (w523:dbl[][])
            "TOBA appended" <- w523
            n157 = case shown="\"Average 15 to 20\", Default" "Temp. Channel selector" {
              tunnel: w559 -> [w629 w631 w634 w637 w640 w643 w646 w649 w656]
              tunnel: [w627 w630 w633 w636 w639 w642 w645 w648 w651] -> w569
              frame "Channel 15" {
                n158 = Index Array(array=w629, index=14) -> (element=w627:dbl)
              }
              frame "Channel 16" {
                n159 = Index Array(array=w631, index=15) -> (element=w630:dbl)
              }
              frame "Channel 17" {
                n160 = Index Array(array=w634, index=16) -> (element=w633:dbl)
              }
              frame "Channel 18" {
                n161 = Index Array(array=w637, index=17) -> (element=w636:dbl)
              }
              frame "Channel 19" {
                n162 = Index Array(array=w640, index=18) -> (element=w639:dbl)
              }
              frame "Channel 20" {
                n163 = Index Array(array=w643, index=19) -> (element=w642:dbl)
              }
              frame "Channel A" {
                n164 = Index Array(array=w646, index=20) -> (element=w645:dbl)
              }
              frame "Channel B" {
                n165 = Index Array(array=w649, index=21) -> (element=w648:dbl)
              }
              frame "Average 15 to 20", Default {
                w652 = 6 ("length")
                n166 = Array Subset(array=w656, index=14, length=w652) -> (w654:dbl[])
                n167 = Add Array Elements(numeric array=w654) -> (sum=w653:dbl)
                n168 = Divide(x=w653, y=w652) -> (x/y=w651:dbl)
              }
            }
            n169 = case shown="\"Channel 17\", Default" "Temperature Channel selector" {
              tunnel: w523 -> [w574 w577 w580 w583 w586 w589 w592 w595]
              tunnel: [w573 w576 w579 w582 w585 w588 w591 w594] -> w556
              frame "Channel 15" {
                n170 = Index Array(array=w574, index (col)=14) -> (element=w573:dbl[])  [unwired: 1 in]
              }
              frame "Channel 16" {
                n171 = Index Array(array=w577, index (col)=15) -> (element=w576:dbl[])  [unwired: 1 in]
              }
              frame "Channel 17", Default {
                n172 = Index Array(array=w580, index (col)=16) -> (element=w579:dbl[])  [unwired: 1 in]
              }
              frame "Channel 18" {
                n173 = Index Array(array=w583, index (col)=17) -> (element=w582:dbl[])  [unwired: 1 in]
              }
              frame "Channel 19" {
                n174 = Index Array(array=w586, index (col)=18) -> (element=w585:dbl[])  [unwired: 1 in]
              }
              frame "Channel 20" {
                n175 = Index Array(array=w589, index (col)=19) -> (element=w588:dbl[])  [unwired: 1 in]
              }
              frame "Channel A" {
                n176 = Index Array(array=w592, index (col)=20) -> (element=w591:dbl[])  [unwired: 1 in]
              }
              frame "Channel B" {
                n177 = Index Array(array=w595, index (col)=21) -> (element=w594:dbl[])  [unwired: 1 in]
              }
            }
            n178 = for {
              N: 22 -> [_]
              tunnel: w539 -> [w661]
              tunnel: [w660] -> w571 mode=indexing
              tunnel: w523 -> [w659]
              i -> [w658]
              n179 = Index Array(array=w659, index (col)=w658) -> (element=w657:dbl[])  [unwired: 1 in]
              n180 = Bundle(w661, w657) -> (w660:cluster{timestamp[], dbl[]})  [unwired: 1 in]
            }
            "Temperature" <- w571
            n181 = Index Array(array=w523, index (col) #1=23 ("disabled index (col)"), index (col) #2=24 ("index (col)"), index (col) #3=25 ("index (col)"), index (col) #4=26 ("index (col)"), index (col) #5=22 ("index (col)")) -> (element #1=w538:dbl[], element #2=w551:dbl[], element #3=w550:dbl[], element #4=w531:dbl[], element #5=w541:dbl[])  [unwired: 5 in]
            n182 = Index Array(array=w559, index=23) -> (element=w560:dbl)
            n183 = Bundle(w556, w538) -> (w555:cluster{dbl[], dbl[]})  [unwired: 1 in]
            n184 = Bundle("Waveform"=w569, "Waveform"=w560) -> (w568:cluster{"Waveform":dbl, "Waveform":dbl})  [unwired: 1 in]
            n185 = Bundle(w539, w538) -> (w549:cluster{timestamp[], dbl[]})  [unwired: 1 in]
            n186 = Bundle(w539, w551) -> (w548:cluster{timestamp[], dbl[]})  [unwired: 1 in]
            n187 = Bundle(w539, w550) -> (w547:cluster{timestamp[], dbl[]})  [unwired: 1 in]
            n188 = Bundle(w539, w531) -> (w544:cluster{timestamp[], dbl[]})  [unwired: 1 in]
            n189 = Bundle(w539, w541) -> (w540:cluster{timestamp[], dbl[]})  [unwired: 1 in]
            n190 = Build Array(w568) -> (→"Phase Diagram":cluster{"Waveform":dbl, "Waveform":dbl}[])
            n191 = Build Array(w555) -> (→"Historical Large Phase Diagram":cluster{dbl[], dbl[]}[])
            n192 = Build Array(w549, w548, w547) -> (→"Pressure":cluster{timestamp[], dbl[]}[])
            n193 = Build Array(w544) -> (→"Flow (SLPM)":cluster{timestamp[], dbl[]}[])
            n194 = Build Array(w540) -> (→"Heater power (%)" →"Heater power (%) 2":cluster{timestamp[], dbl[]}[])
            n195 = case shown="\"Average 15 to 20\", Default" "Temperature Channel selector" {
              tunnel: w559 -> [w599 w601 w604 w607 w610 w613 w616 w619 w626]
              tunnel: [w597 w600 w603 w606 w609 w612 w615 w618 w621] -> w564
              frame "Channel 15" {
                n196 = Index Array(array=w599, index=14) -> (element=w597:dbl)
              }
              frame "Channel 16" {
                n197 = Index Array(array=w601, index=15) -> (element=w600:dbl)
              }
              frame "Channel 17" {
                n198 = Index Array(array=w604, index=16) -> (element=w603:dbl)
              }
              frame "Channel 18" {
                n199 = Index Array(array=w607, index=17) -> (element=w606:dbl)
              }
              frame "Channel 19" {
                n200 = Index Array(array=w610, index=18) -> (element=w609:dbl)
              }
              frame "Channel 20" {
                n201 = Index Array(array=w613, index=19) -> (element=w612:dbl)
              }
              frame "Channel A" {
                n202 = Index Array(array=w616, index=20) -> (element=w615:dbl)
              }
              frame "Channel B" {
                n203 = Index Array(array=w619, index=21) -> (element=w618:dbl)
              }
              frame "Average 15 to 20", Default {
                w622 = 6 ("length")
                n204 = Array Subset(array=w626, index=14, length=w622) -> (w624:dbl[])
                n205 = Add Array Elements(numeric array=w624) -> (sum=w623:dbl)
                n206 = Divide(x=w623, y=w622) -> (x/y=w621:dbl)
              }
            }
            n207 = Reverse 1D Array(array=w538) -> (reversed array=w537:dbl[])
            n208 = Reverse 1D Array(array=w531) -> (reversed array=w533:dbl[])
            n209 = Array Subset(array=w537, length="N samples") -> (w526:dbl[])  [unwired: 1 in]
            n210 = Array Subset(array=w533, length="N samples") -> (w528:dbl[])  [unwired: 1 in]
            n211 = Array Size(array=w528) -> (size(s)=w527:i32)
            n212 = Array Size(array=w526) -> (size(s)=w525:i32)
            n213 = Add Array Elements(numeric array=w528) -> (sum=w532:dbl)
            n214 = Add Array Elements(numeric array=w526) -> (sum=w536:dbl)
            n215 = Bundle("Waveform"=w564, "Waveform"=w560) -> (w565:cluster{"Waveform":dbl, "Waveform":dbl})  [unwired: 1 in]
            n216 = Divide(x=w532, y=w527) -> (x/y=→"Average Flow (SLPM)":dbl)
            n217 = Divide(x=w536, y=w525) -> (x/y=→"Moving average Det. P":dbl)
            n218 = Build Array(w565) -> (→"Large Phase Diagram":cluster{"Waveform":dbl, "Waveform":dbl}[])
          }
          frame #5 {
            # "Temperatures (20),      NI Box;\nTemperatures (4),  Lakeshore;\nHeater Power,       Lakeshore;\nPressures (4),               NI Box;\nSetpoint,               Lakeshore;\nCurrent time (s)               ---   ;\nCycle time (s)                   ---   ;"
            # "Saving data"
            n219 = Get Date/Time In Seconds() -> (seconds since 1Jan1904=w675:timestamp)
            n220 = To Double Precision Float(number=w675) -> (double precision float=w674:dbl)
            n221 = Build Array (concatenate)(w677, w676, w674, w673, w672) -> (w671:dbl[])
            n222 = Get Date/Time String() -> (date string=w665:string)  [unwired: 3 in, 1 out]
            n223 = Build Path(base path=path "D:/Log_data/SC_LOG", name or relative path=w665) -> (appended path=w664:path)
            n224 = Format Date/Time String() -> (date/time string=w669:string)  [unwired: 3 in]
            n225 = Array To Spreadsheet String(array=w671, 3:"%.3f" ("format string")) -> (spreadsheet string=w667:string)  [unwired: 1 in]
            n226 = Concatenate Strings(w669, "\t", w667) -> (w663:string)
            n227 = call <vilib>:"Write Spreadsheet String.vi"("append to file? (new file:F)"=TRUE, "spreadsheet string"=w663, "file path (dialog if empty)"=w664) -> ()  [unwired: 7 in, 2 out]
          }
          frame #6 {
            # "Alarm conditions (Temp)"
            # "NI mod2 & 3 status go here"
            # "Check alarms and UPS"
            n228 = Unbundle By Name(w706) -> ("error out.status"=w703:bool)
            "LakeShore status" <- w703
            n229 = Unbundle By Name(w708) -> ("error out.status"=w702:bool)
            "CAEN 1 status" <- w702
            n230 = Unbundle By Name(w707) -> ("error out.status"=w701:bool)
            "CAEN 2 status" <- w701
            n231 = Unbundle By Name(w704) -> ("error out.status"=w700:bool)
            "NI mod1 (P) status" <- w700
            n232 = Index Array(array=w689, index=23) -> (element=w695:dbl)
            n233 = Build Array(w703, w702, w701, w700) -> (w699:bool[])
            n234 = Or Array Elements(Boolean array=w699) -> (logical OR=→"Comm. status":bool)
            n235 = Greater?(x=w695, y="Overpressure threshold") -> (0:w693:bool)
            n236 = Less?(x=w695, y="Underpressure threshold") -> (x < y?=w692:bool)
            n237 = Or(x=w693, y=w692) -> (x .or. y?=w691:bool)
            n238 = And(x="Detector P", y=w691) -> ()  [unwired: 1 out]
            n239 = Array Subset(array=w689, index=14, length=6) -> (w686:dbl[])
            n240 = Build Array("T 15", "T 16", "T 17", "T 18", "T 19", "T 20") -> (w678:bool[])
            n241 = for {
              tunnel: w686 -> [w713] mode=indexing
              tunnel: [w710] -> w685 mode=indexing
              tunnel: w678 -> [w709] mode=indexing
              n242 = Greater?(x=w713, y="High Temp threshold") -> (0:w712:bool)
              n243 = Less?(x=w713, y="Low Temp threshold") -> (x < y?=w711:bool)
              n244 = Or(x=w712, y=w711) -> (x .or. y?=w710:bool)
              n245 = And(x=w709, y=w710) -> ()  [unwired: 1 out]
            }
            n246 = Index Array(array=w685) -> ()  [unwired: 1 in, 1 out]
          }
        }
        n247 = Decrement(x="Cycles to execute") -> (x-1=w131:dbl)
        n248 = Greater?(x=w143, y=w131) -> ()  [unwired: 1 out]
        n249 = Or(x=FALSE, y="stop") -> (x .or. y?=w146:bool)
      }
      "TOBA tester" <- w110
    }
    frame True {
    }
  }
  n250 = Array Size(array=w20) -> (size(s)=w23:i32)
  n251 = flat-sequence {
    tunnel: w7 -> [w742]
    tunnel: w3 -> [w733]
    tunnel: w2 -> [w730]
    tunnel: w1 -> [w725]
    frame #0 {
      w738 = u16 2 items=["1"=1, "2"=2] ("Heater Output (1:1)")
      w739 = u16 0 items=["Off", "Low (On)", "Medium", "High"] ("Range (0:Off)")
      # "Turn off heater, shutdown COM"
      # "Error Handling and Post-Processing (EHaPP)"
      n252 = Unbundle(w742) -> ("VISA resource name out"=w741:refnum<visa-resource-name>, "error out"=w740:errorcluster)
      n253 = Unbundle(w733) -> ("VISA resource name out"=w732:refnum<visa-resource-name>, "error out"=w731:errorcluster)
      n254 = Unbundle(w730) -> ("VISA resource name out"=w729:refnum<visa-resource-name>, "error out"=w728:errorcluster)
      n255 = Unbundle(w725) -> ("task out"=w724:refnum<k21>, "error out"=w723:errorcluster)
      n256 = call <instrlib>:"Configure Output Range and Manual Value.vi"("VISA resource name"=w741, "Heater Output (1:1)"=w738, "Range (0:Off)"=w739, "Manual Output (0.00 %)"=0.0, "error in (no error)"=w740) -> ("VISA resource name out"=w736:refnum<visa-resource-name>, "error out"=w735:errorcluster)  [unwired: 9 in]
      n257 = call <instrlib>:"Close.vi"("error in (no error)"=w731, "VISA resource name"=w732) -> ("error out"=w727:errorcluster)  [unwired: 9 in]
      n258 = call <instrlib>:"Close.vi"("error in (no error)"=w728, "VISA resource name"=w729) -> ("error out"=w726:errorcluster)  [unwired: 9 in]
      n259 = call <vilib>:"DAQmx Clear Task.vi"("task in"=w724, "error in"=w723) -> ("error out"=w722:errorcluster)  [unwired: 13 in]
      n260 = call <instrlib>:"Close.vi"("error in (no error)"=w735, "VISA resource name"=w736) -> ("error out"=w734:errorcluster)  [unwired: 9 in]
      n261 = call <vilib>:"Simple Error Handler.vi"("error in (no error)"=w734) -> ()  [unwired: 4 in, 5 out]
      n262 = call <vilib>:"Simple Error Handler.vi"("error in (no error)"=w727) -> ()  [unwired: 4 in, 5 out]
      n263 = call <vilib>:"Simple Error Handler.vi"("error in (no error)"=w726) -> ()  [unwired: 4 in, 5 out]
      n264 = call <vilib>:"Simple Error Handler.vi"("error in (no error)"=w722) -> ()  [unwired: 4 in, 5 out]
    }
  }
  n265 = Decrement(x=w23) -> (x-1=w22:i32)
  n266 = Index Array(array=w20, index=w22) -> (element=w21:timestamp)
  n267 = Index Array(array=w20, index=1) -> (element=w18:timestamp)
  n268 = To Double Precision Float(number=w21) -> (double precision float=w17:dbl)
  n269 = To Double Precision Float(number=w18) -> (double precision float=w16:dbl)
  n270 = Subtract(x=w17, y=w16) -> ()  [unwired: 1 out]
  "Started up?" <- w12
